vi "SLL DE Check AO Values within limit.vi"(7 "Display Dialog":bool, 8 "AO Min Values":dbl, 9 "AO Max Values":dbl, 10 "AO Value":dbl, 11 "AO Channel Name":T1) -> (2 "value":dbl)   [LabVIEW 2013]
uses:
  Controls/SLL DE List of Analog Outputs.ctl
  Instance           1 43Saved   SLL DE Check AO Values within limit .vi
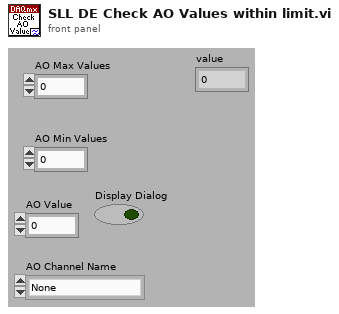
[diagram p1: front panel]
types:
  T1 = typedef "SLL DE List of Analog Outputs.ctl" = enum16{"None"}
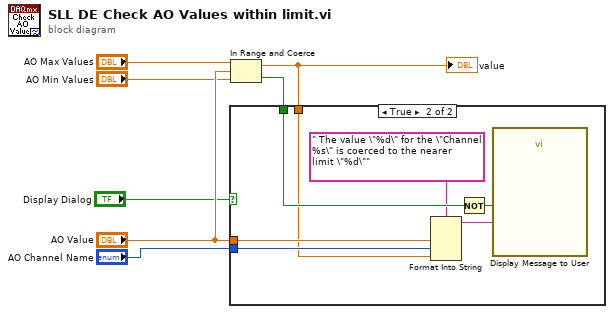
[diagram p0: block diagram]
diagram:
  n1 = In Range and Coerce(upper limit="AO Max Values", x="AO Value", lower limit="AO Min Values") -> (coerced(x)=w4:dbl, In Range?=w7:bool)
  "value" <- w4
  n2 = case shown="True" "Display Dialog" {
    tunnel: w7 -> [_ w14]
    tunnel: "AO Channel Name" -> [_ w13]
    tunnel: "AO Value" -> [_ w9]
    tunnel: w4 -> [_ w8]
    frame False {
    }
    frame True {
      n3 = Format Into String(format string=" The value \"%d\" for the \"Channel %s\" is coerced to the nearer limit \"%d\"", w9, w13, w8) -> (resulting string=w11:string)  [unwired: 2 in, 1 out]
      n4 = Not(x=w14) -> (.not. x?=w10:bool)
      n5 = call "Display Message to User"("Enable"=w10, "Message"=w11) -> ()  [unwired: 8 in, 2 out]
    }
  }
